vi "RoboLogUI.vi"(4 "terminalBufferLength(lines)":u32, 6 "Notifiers":T1, 8 "DefaultLocalPath":path, 9 "remoteLoggerPort":u16, 10 "ConnectionData":T2, 11 "remotePath":string) -> ()   [LabVIEW 2015]
uses:
  General/RemoteFiles/connectionData.ctl
  LoggerViewer/src/LoggerMonitorControlData.ctl
panel:
  out "connectedToLogger":bool caption="Connected to Logger?"
  out "windowName":string
  in  "clearLogBtn":bool
  in  "Remote Log Directory":string
  in  "refreshBtn":bool
  out "Logger Console":string
  in  "viewBtn":bool
  in  "copyBtn":bool
  in  "deleteBtn":bool
  in  "Remote Logs":string(tree)
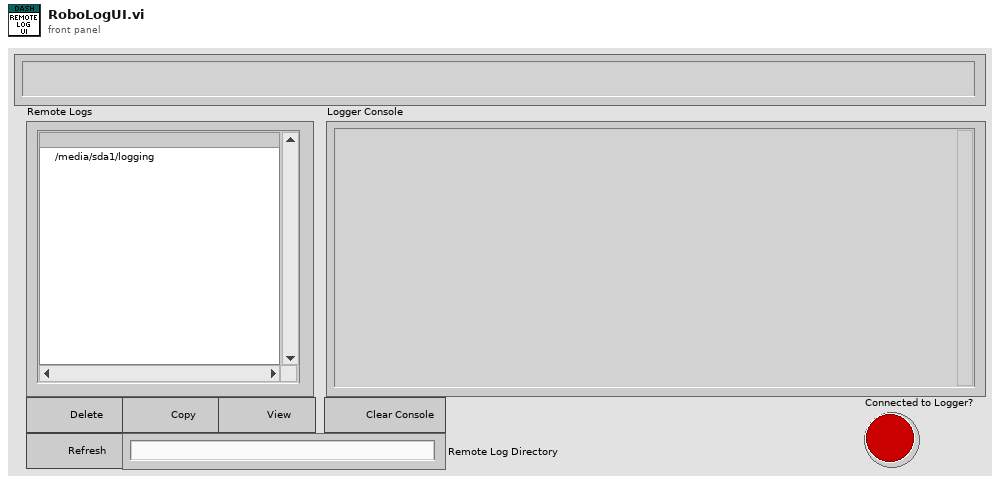
[diagram p1: front panel]
types:
  T1 = cluster{"WindowNotifier":refnum<notifier>, "Stop_Notifier":refnum<notifier>}
  T2 = typedef "connectionData.ctl" = cluster{"host":string, "user":string, "password":string, "port":u16}
  T3 = typedef "LoggerMonitorControlData.ctl" = cluster{"clearLogBtn":refnum<vi>, "terminalBufferLength(lines)":i32, "remoteLoggerPort":u16, "Remote Log Directory":refnum<vi>, "refreshBtn":refnum<vi>, "Logger Console":refnum<vi>, "ConnectionData":T2, "remotePath":refnum<vi>, "viewBtn":refnum<vi>, "copyBtn":refnum<vi>, "deleteBtn":refnum<vi>, "Remote Logs":refnum<vi>, "windowName":refnum<vi>, "DefaultLocalPath":path, "WindowNotifier":refnum<notifier>, "Stop_Notifier":refnum<notifier>, "connectedToLogger":refnum<vi>}
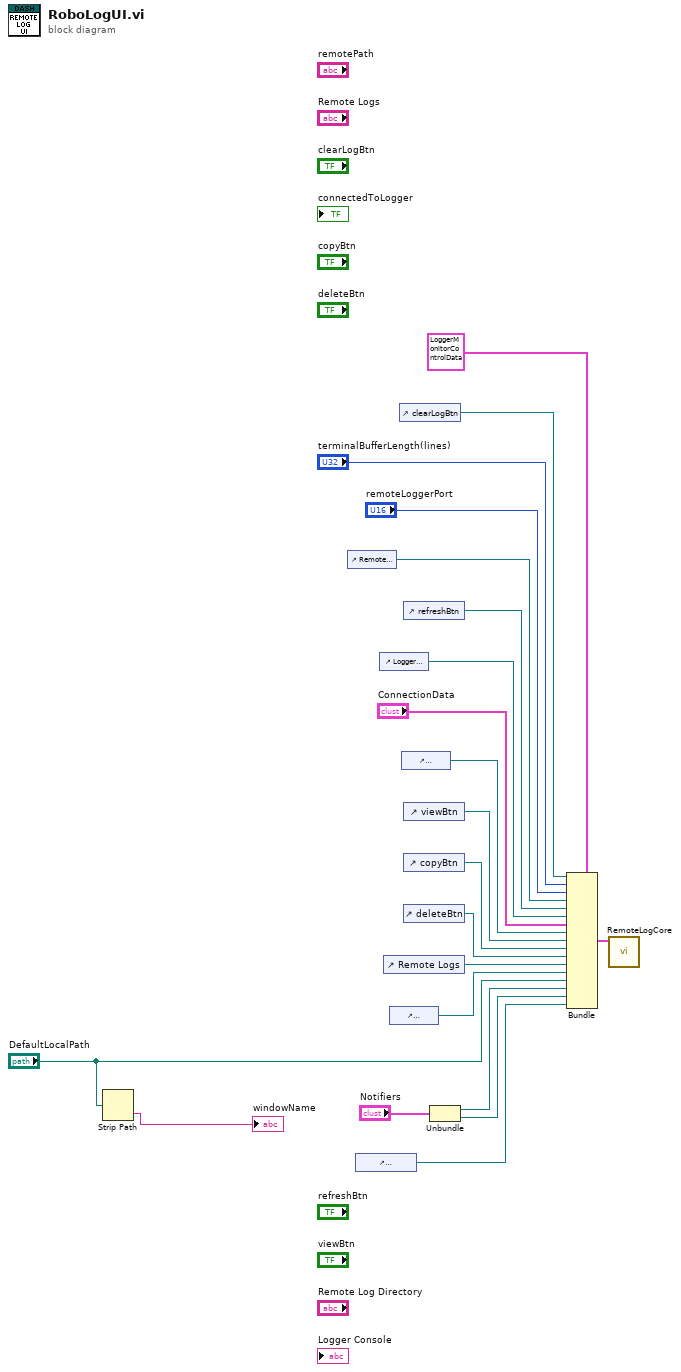
[diagram p0: block diagram]
diagram:
  n1 = Strip Path(path="DefaultLocalPath") -> (name=→"windowName":string)  [unwired: 1 out]
  n2 = control-ref of="Remote Log Directory"() -> (w20:refnum<vi>)
  n3 = control-ref of="connectedToLogger"() -> (w4:refnum<vi>)
  n4 = control-ref of="Logger Console"() -> (w18:refnum<vi>)
  n5 = control-ref of="Remote Logs"() -> (w13:refnum<vi>)
  n6 = control-ref of="windowName"() -> (w12:refnum<vi>)
  n7 = control-ref of="clearLogBtn"() -> (w21:refnum<vi>)
  n8 = control-ref of="remotePath"() -> (w17:refnum<vi>)
  n9 = control-ref of="refreshBtn"() -> (w19:refnum<vi>)
  n10 = control-ref of="viewBtn"() -> (w16:refnum<vi>)
  n11 = control-ref of="copyBtn"() -> (w15:refnum<vi>)
  n12 = control-ref of="deleteBtn"() -> (w14:refnum<vi>)
  n13 = Unbundle("Notifiers") -> ("WindowNotifier"=w10:refnum<notifier>, "Stop_Notifier"=w9:refnum<notifier>)
  n14 = Bundle(cluster=T3 {"clearLogBtn"=refnum, "terminalBufferLength(lines)"=0, "remoteLoggerPort"=0, "Remote Log Directory"=refnum, "refreshBtn"=refnum, "Logger Console"=refnum, "ConnectionData"={"host"="", "user"="", "password"="", "port"=0}, "remotePath"=refnum, "viewBtn"=refnum, "copyBtn"=refnum, "deleteBtn"=refnum, "Remote Logs"=refnum, "windowName"=refnum, "DefaultLocalPath"=path "", "WindowNotifier"=refnum, "Stop_Notifier"=refnum, "connectedToLogger"=refnum} ("LoggerMonitorControlData"), "clearLogBtn"=w21, "terminalBufferLength(lines)"="terminalBufferLength(lines)", "remoteLoggerPort"="remoteLoggerPort", "Remote Log Directory"=w20, "refreshBtn"=w19, "Logger Console"=w18, "ConnectionData"="ConnectionData", "remotePath"=w17, "viewBtn"=w16, "copyBtn"=w15, "deleteBtn"=w14, "Remote Logs"=w13, "windowName"=w12, "DefaultLocalPath"="DefaultLocalPath", "WindowNotifier"=w10, "Stop_Notifier"=w9, "connectedToLogger"=w4) -> (w7:T3)
  n15 = call "RemoteLogCore.vi"("LoggerMonitorControlData"=w7) -> ()  [unwired: 11 in]
